vi "DirettoreOpen.vi"(8 "MatrixFIFODepth":i32, 9 "TriggerFIFODepth":u32) -> (0 "ErrorOut":errorcluster, 3 "FPGAReference":refnum<k20>)   [LabVIEW 2012]
uses:
  <vilib>/FPGAPlugInAG/PCIe-7852R/niLvFpga_Open_PCIe-7852R.vi
  <vilib>/rvi/interface/common/dynamic/niFpgaDynamicAddResources.vi
  <vilib>/Utility/error.llb/Error Cluster From Error Code.vi
  <vilib>/FPGAPlugInAG/Dynamic/niLvFpga_Reset_Dynamic.vi
  <vilib>/rvi/interface/nirviOpenFPGA/nirviOpenFPGA.xnode
  FPGA Bitfiles/Direttore.lvbitx
  <vilib>/rvi/interface/nirviMethod/nirviMethod.xnode
  <vilib>/rvi/errors/niLvFpgaMergeErrorWithErrorCode.vi
  <vilib>/FPGAPlugInAG/Dynamic/niLvFpga_ConfigureFifo_Dynamic.vi
panel:
  out "ActualDepthPlayTriggerFIFO":u32
  out "ActualDepthOutPutMatrixFIFO":u32
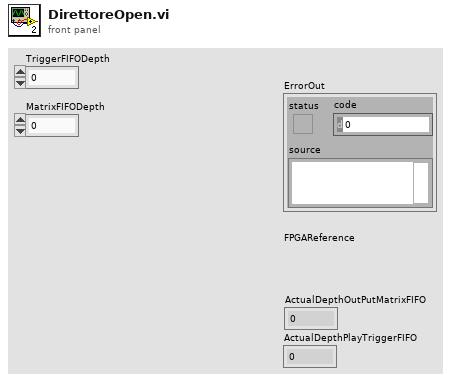
[diagram p1: front panel]
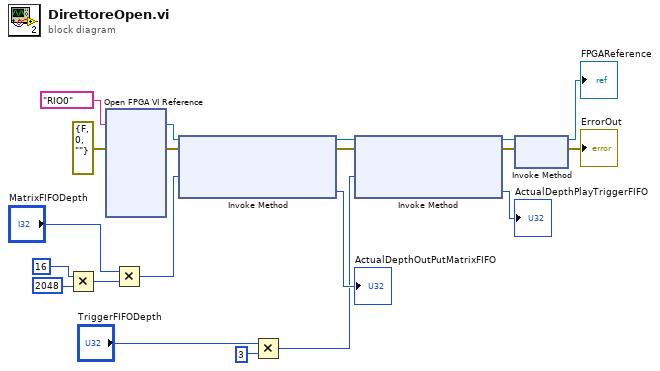
[diagram p0: block diagram]
diagram:
  n1 = Multiply(x=16, y=2048) -> (x*y=w10:i32)
  n2 = xnode "Open FPGA VI Reference"("error in"=errorcluster {"status"=FALSE, "code"=0, "source"=""}, "resource name"=tag "RIO0") -> ("FPGA VI Reference Out"=w16:refnum<k20>, "error out"=w13:errorcluster)
  n3 = Multiply(x="MatrixFIFODepth", y=w10) -> (x*y=w9:i32)
  n4 = xnode "Invoke Method"("FPGA VI Reference In"=w16, "error in"=w13, "Requested Depth"=w9) -> ("FPGA VI Reference Out"=w12:refnum<k20>, "error out"=w11:errorcluster, "Actual Depth"=→"ActualDepthOutPutMatrixFIFO":u32)
  n5 = Multiply(x="TriggerFIFODepth", y=u32 3) -> (x*y=w7:u32)
  n6 = xnode "Invoke Method"("FPGA VI Reference In"=w12, "error in"=w11, "Requested Depth"=w7) -> ("FPGA VI Reference Out"=w2:refnum<k20>, "error out"=w3:errorcluster, "Actual Depth"=→"ActualDepthPlayTriggerFIFO":u32)
  n7 = xnode "Invoke Method"("FPGA VI Reference In"=w2, "error in"=w3) -> ("FPGA VI Reference Out"=→"FPGAReference":refnum<k20>, "error out"=→"ErrorOut":errorcluster)
